vi "SolvePnP-USAC.vi"(6 "Camera Parameters":T7, 7 "USAC Params (Default: OpenCV Defaults)":refnum<class "USAC Params.lvclass">, 8 "error in (no error)":errorcluster, 11 "Point Correspondence Set":T1) -> (0 "error out":errorcluster, 3 "Pose":T4, 4 "Inliers":i32[](array[numeric]))   [LabVIEW 2020, in "g_ar_toolkit.ar.lvlib"]
uses:
  g_ar_toolkit.ar.lvlib
  rvec.ctl
  g_ar_toolkit.common/tvec.ctl
  Pose.ctl
  g_ar_toolkit.common/g_ar_toolkit.common.lvlib
  USAC Params/USAC Params.lvclass
  g_ar_toolkit.common/Camera Matrix.ctl
  g_ar_toolkit.common/Camera Distortion Coefficients.ctl
  g_ar_toolkit.common/Camera Parameters.ctl
  g_ar_toolkit.common/Image Point (Float).ctl
  g_ar_toolkit.common/Object Point (Float).ctl
  Point Correspondence Set.ctl
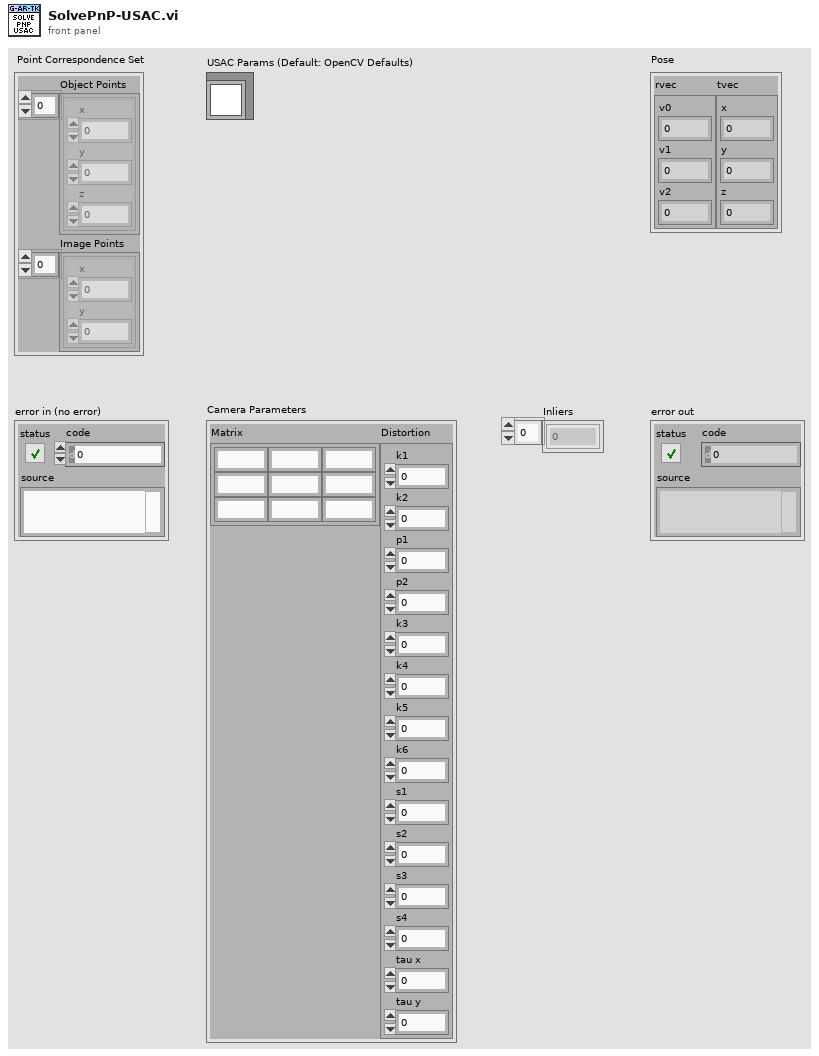
[diagram p1: front panel]
types:
  T1 = typedef "g_ar_toolkit.ar.lvlib/Point Correspondence Set.ctl" = cluster{"Object Points":T2[], "Image Points":T3[]}
  T2 = typedef "g_ar_toolkit.common.lvlib/Object Point (Float).ctl" = cluster{"x":dbl, "y":dbl, "z":dbl}
  T3 = typedef "g_ar_toolkit.common.lvlib/Image Point (Float).ctl" = cluster{"x":dbl, "y":dbl}
  T4 = typedef "g_ar_toolkit.ar.lvlib/Pose.ctl" = cluster{"rvec":T5, "tvec":T6}
  T5 = typedef "g_ar_toolkit.ar.lvlib/rvec.ctl" = cluster{"v0":dbl, "v1":dbl, "v2":dbl}
  T6 = typedef "g_ar_toolkit.ar.lvlib/tvec.ctl" = cluster{"x":dbl, "y":dbl, "z":dbl}
  T7 = typedef "g_ar_toolkit.common.lvlib/Camera Parameters.ctl" = cluster{"Matrix":T8, "Distortion":T9}
  T8 = typedef "g_ar_toolkit.common.lvlib/Camera Matrix.ctl" = cluster{"m 0,0":dbl, "m 0,1":dbl, "m 0,2":dbl, "m 1,0":dbl, "m 1,1":dbl, "m 1,2":dbl, "m 2,0":dbl, "m 2,1":dbl, "m 2,2":dbl}
  T9 = typedef "g_ar_toolkit.common.lvlib/Camera Distortion Coefficients.ctl" = cluster{"k1":dbl, "k2":dbl, "p1":dbl, "p2":dbl, "k3":dbl, "k4":dbl, "k5":dbl, "k6":dbl, "s1":dbl, "s2":dbl, "s3":dbl, "s4":dbl, "tau x":dbl, "tau y":dbl}
  T10 = typedef "g_ar_toolkit.ar.lvlib/USAC Params.lvclass/Parameters.ctl" = cluster{"Confidence":dbl, "Threshold":dbl, "Final Polisher Iterations":i32, "Local Optimization Iterations":u16, "Local Optimization Sample Size":u16, "Max Iterations":u16, "Random Generator State":i32, "Final Polisher":T11, "Local Optimization Method":T12, "Neighbor Search Method":T13, "Sampler":T14, "Score":T15, "Is Parallel":bool}
  T11 = typedef "g_ar_toolkit.ar.lvlib/USAC Params.lvclass/Polishing Methods.ctl" = enum8{"NONE", "LSQ", "MAGSAC", "COV"}
  T12 = typedef "g_ar_toolkit.ar.lvlib/USAC Params.lvclass/Local Optimization Methods.ctl" = enum8{"NULL", "INNER_LO", "INNER_AND_ITER_LO", "GC", "SIGMA"}
  T13 = typedef "g_ar_toolkit.ar.lvlib/USAC Params.lvclass/Neighbor Search Methods.ctl" = enum8{"FLANN_KNN", "GRID", "FLANN_RADIUS"}
  T14 = typedef "g_ar_toolkit.ar.lvlib/USAC Params.lvclass/Sampling Methods.ctl" = enum8{"UNIFORM", "PROGRESSIVE_NAPSAC", "NAPSAC", "PROSAC"}
  T15 = typedef "g_ar_toolkit.ar.lvlib/USAC Params.lvclass/Score Methods.ctl" = enum8{"RANSAC", "MSAC", "MAGSAC", "LMEDS"}
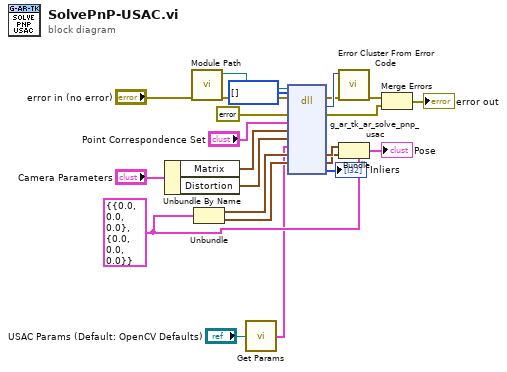
[diagram p0: block diagram]
diagram:
  w20 = T4 {"rvec"={"v0"=0.0, "v1"=0.0, "v2"=0.0}, "tvec"={"x"=0.0, "y"=0.0, "z"=0.0}} ("Pose (Estimate)")
  n1 = Unbundle By Name("Camera Parameters") -> ("Matrix"=w10:T8, "Distortion"=w9:T9)
  n2 = call "Module Path.vi"("error in (no error)"="error in (no error)") -> ("error out"=w16:errorcluster, "Path"=w17:path)  [unwired: 9 in]
  n3 = Unbundle(w20) -> ("rvec"=w8:T5, "tvec"=w7:T6)
  n4 = call "Get Params.vi"("USAC Params in"="USAC Params (Default: OpenCV Defaults)") -> ("Parameters"=w2:T10)
  n5 = dll-call lib="?" fn="g_ar_tk_ar_solve_pnp_usac" ("g_ar_toolkit.*.*:g_ar_tk_image_copy")(path in=w17, error in=w16, "error_cluster"=errorcluster {"status"=FALSE, "code"=0, "source"=""} ("error constant"), "corespondence"="Point Correspondence Set", "camera_matrix"=w10, "camera_distortion"=w9, "usac_parameters"=w2, "rvec"=w8, "tvec"=w7, "inliers"=i32[] []) -> (error out=w11:errorcluster, "MgErr"=w12:i32, "error_cluster"=w15:errorcluster, "rvec"=w6:T5, "tvec"=w5:T6, "inliers"=→"Inliers":i32[])  [unwired: 5 in, 1 out]
  n6 = call <vilib>:"Error Cluster From Error Code.vi"("error in (no error)"=w11, "error code (0)"=w12) -> ("error out"=w13:errorcluster)  [unwired: 7 in]
  n7 = Bundle(cluster=w20, "rvec"=w6, "tvec"=w5) -> (→"Pose":T4)
  n8 = Merge Errors(w13, w15) -> (→"error out":errorcluster)
